vi "Rinocloud_HTTP_ancestors.vi"(4 "id":string, 7 "Tree Ref in":refnum<vi>) -> (0 "body":string, 1 "headers":string, 2 "last ID":string, 3 "Tree Ref out":refnum<vi>)   [LabVIEW 2013]
uses:
  Rinocloud_global_variable.vi
  <vilib>/httpClient/POSTBuffer.vi
  <vilib>/LVH/i3 JSON/JSON Parsing/Get Array Value at Index Files/Get Array Value at Index - Array.vi
  <vilib>/LVH/i3 JSON/JSON Parsing/Get Object Parameter Files/Get Object Parameter - String.vi
  <vilib>/LVH/i3 JSON/JSON Parsing/Get Object Parameter Files/Get Object Parameter - Numeric.vi
  <vilib>/httpClient/LabVIEWHTTPClient.lvlib
  i3 JSON/i3-json.lvlib
panel:
  out "error out":errorcluster
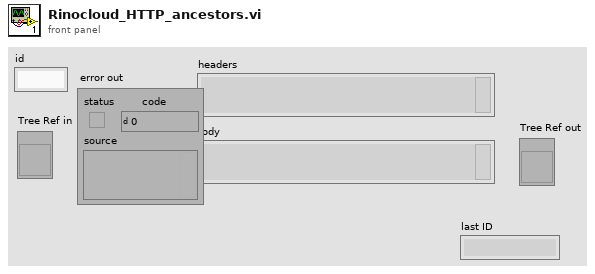
[diagram p1: front panel]
types:
  T1 = typedef "LabVIEWHTTPClient.lvlib/ClientHandle.ctl" = refnum<k1>
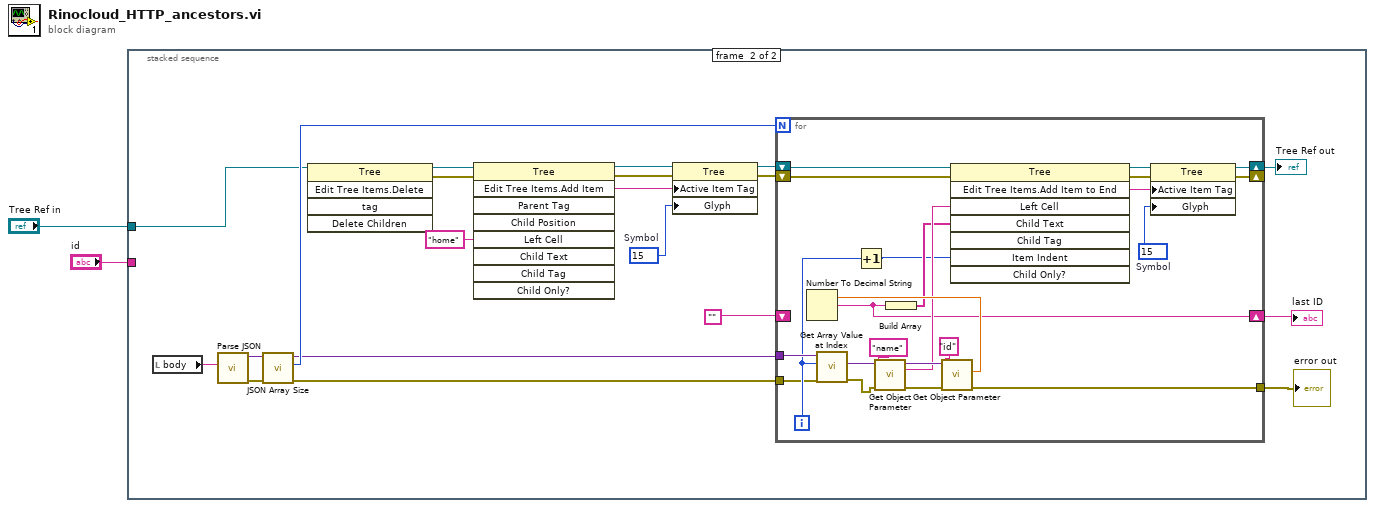
[diagram p0: block diagram]
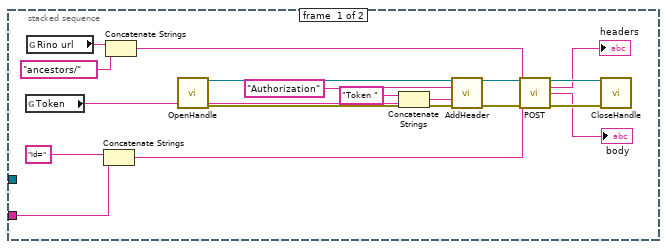
[diagram p2: hidden frame]
diagram:
  n1 = stacked-sequence {
    tunnel: "id" -> [w6 _]
    tunnel: "Tree Ref in" -> [_ w35]
    frame #0 {
      n2 = global read "Rinocloud_global_variable.vi" "Token"() -> (w12:string)
      n3 = global read "Rinocloud_global_variable.vi" "Rino url"() -> (w18:string)
      n4 = Concatenate Strings("id=" ("value"), w6) -> (w3:string)
      n5 = Concatenate Strings(w18, "ancestors/" ("Combo Box 2")) -> (w20:string)
      n6 = call <vilib>:"OpenHandle.vi"() -> ("client handle out"=w16:T1, "error out"=w13:errorcluster)  [unwired: 14 in]
      n7 = Concatenate Strings("Token " ("value"), w12) -> (w14:string)
      n8 = call <vilib>:"AddHeader.vi"("client handle"=w16, "header"="Authorization" ("url"), "value"=w14, "error in (no error)"=w13) -> ("client handle out"=w9:T1, "error out"=w8:errorcluster)  [unwired: 10 in]
      n9 = call-poly <vilib>:"POST.vi"("client handle"=w9, "url"=w20, "buffer"=w3, "error in (no error)"=w8) -> ("client handle out"=w11:T1, "headers"=→"headers":string, "body"=→"body":string, "error out"=w10:errorcluster)  [unwired: 8 in]
      n10 = call <vilib>:"CloseHandle.vi"("client handle"=w11, "error in (no error)"=w10) -> ()  [unwired: 13 in, 1 out]
    }
    frame #1 {
      w25 = 15  # Symbol
      n11 = local read "body"() -> (w40:string)
      n12 = call <vilib>:"Parse JSON.vi"("JSON String"=w40) -> ("error out"=w39:errorcluster, "JSON Tree"=w38:variant)  [unwired: 7 in, 2 out]
      n13 = call <vilib>:"JSON Array Size.vi"("error in (no error)"=w39, "JSON Tree In (JSON Array)"=w38) -> ("error out"=w24:errorcluster, "Array Size"=w37:i32, "JSON Tree Passthrough (JSON Array)"=w36:variant)  [unwired: 7 in]
      n14 = invoke class="Tree" method="Edit Tree Items.Delete"(reference=w35) -> (reference out=w33:refnum<vi>, error out=w32:errorcluster)  [unwired: 4 in, 3 out]
      n15 = invoke class="Tree" method="Edit Tree Items.Add Item"(reference=w33, error in=w32, "Left Cell"="home" ("Left Cell String")) -> (reference out=w30:refnum<vi>, error out=w28:errorcluster, "Edit Tree Items:Add Item"=w26:string)  [unwired: 6 in, 6 out]
      n16 = property class="Tree"(reference=w30, error in=w28, "Active Item Tag"=w26, "Glyph"=w25) -> (reference out=w29:refnum<vi>, error out=w27:errorcluster)
      n17 = for {
        N: w37 -> [_]
        tunnel: w36 -> [w62]
        shift-right: [w54] -> w34
        shift-left: w29 -> [w57]
        shift-right: [w53] -> _
        shift-left: w27 -> [w55]
        tunnel: w24 -> [w45]
        shift-right: [w42] -> w21
        shift-left: "" -> [_]
        tunnel: [w41] -> w22
        i -> [w46]
        w48 = 15  # Symbol
        n18 = call-poly <vilib>:"Get Array Value at Index.vi"("error in (no error)"=w45, "Index"=w46, "JSON Tree In (JSON Array)"=w62) -> ("error out"=w44:errorcluster, "JSON Array"=w61:variant)  [unwired: 5 in, 2 out]
        n19 = Increment(x=w46) -> (x+1=w47:i32)
        n20 = call-poly <vilib>:"Get Object Parameter.vi"("error in (no error)"=w44, "Parameter Name"="name", "JSON Tree In (JSON Object)"=w61) -> ("error out"=w43:errorcluster, "String Value"=w50:string, "JSON Tree Out Passthrough"=w59:variant)  [unwired: 5 in, 1 out]
        n21 = call-poly <vilib>:"Get Object Parameter.vi"("error in (no error)"=w43, "Parameter Name"="id", "JSON Tree In (JSON Object)"=w59) -> ("error out"=w41:errorcluster, "Double Value"=w58:dbl)  [unwired: 5 in, 2 out]
        n22 = Number To Decimal String(number=w58) -> (decimal integer string=w42:string)  [unwired: 1 in]
        n23 = Build Array(w42) -> (w49:string[])
        n24 = invoke class="Tree" method="Edit Tree Items.Add Item to End"(reference=w57, error in=w55, "Left Cell"=w50, "Child Text"=w49, "Item Indent"=w47) -> (reference out=w56:refnum<vi>, error out=w52:errorcluster, "Edit Tree Items:Add Item to End"=w51:string)  [unwired: 3 in, 5 out]
        n25 = property class="Tree"(reference=w56, error in=w52, "Active Item Tag"=w51, "Glyph"=w48) -> (reference out=w54:refnum<vi>, error out=w53:errorcluster)
      }
      "Tree Ref out" <- w34
      "error out" <- w22
      "last ID" <- w21
    }
  }
